vi "recordset get field names.vi"(8 "error in (no error)":errorcluster, 11 "recordset in":refnum<k7>) -> (0 "error out":errorcluster, 2 "field names":string[](array[string]), 3 "recordset out":refnum<k7>)   [LabVIEW 2020, in "ADODB.lvlib"]
uses:
  ADODB.lvlib
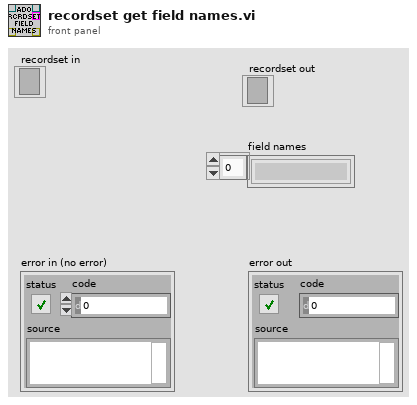
[diagram p1: front panel]
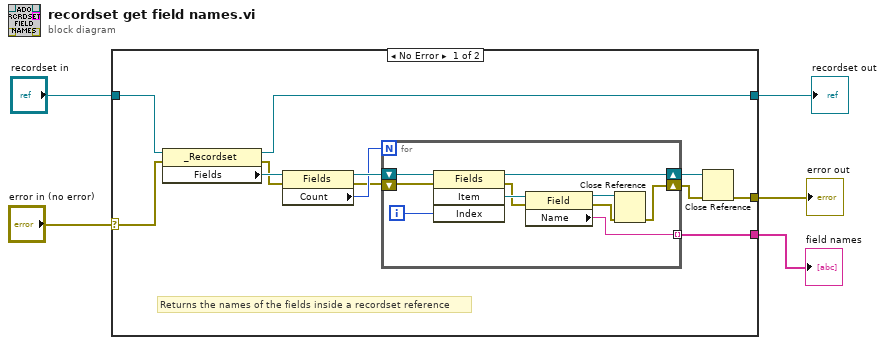
[diagram p0: block diagram]
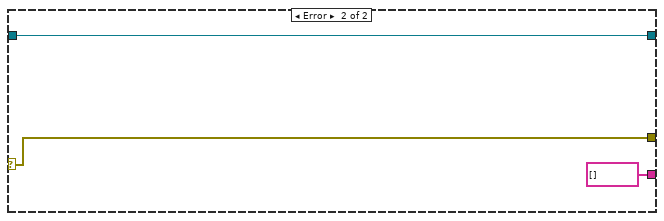
[diagram p2: hidden frame]
diagram:
  n1 = case shown="No Error" "error in (no error)" {
    selector: "error in (no error)" -> [w7 w30]
    tunnel: "recordset in" -> [w17 w28]
    tunnel: [w12 w28] -> w4
    tunnel: [w8 w30] -> w3
    tunnel: [w6 string[] []] -> w1
    frame No Error {
      # "Returns the names of the fields inside a recordset reference"
      n2 = property class="_Recordset"(reference=w17, error in=w7) -> (reference out=w12:refnum<k7>, error out=w11:errorcluster, "Fields"=w16:refnum<k7>)
      n3 = property class="Fields"(reference=w16, error in=w11) -> (reference out=w15:refnum<k7>, error out=w10:errorcluster, "Count"=w14:i32)
      n4 = for {
        N: w14 -> [_]
        tunnel: [w24] -> w6 mode=indexing
        shift-right: [w22] -> w13
        shift-left: w15 -> [w27]
        shift-right: [w18] -> w9
        shift-left: w10 -> [w21]
        i -> [w26]
        n5 = invoke class="Fields" method="Item"(reference=w27, error in=w21, "Index"=w26) -> (reference out=w22:refnum<k7>, error out=w20:errorcluster, "Item"=w25:refnum<k7>)  [unwired: 1 in, 1 out]
        n6 = property class="Field"(reference=w25, error in=w20) -> (reference out=w23:refnum<k7>, error out=w19:errorcluster, "Name"=w24:string)
        n7 = Close Reference(reference=w23, error in (no error)=w19) -> (error out=w18:errorcluster)
      }
      n8 = Close Reference(reference=w13, error in (no error)=w9) -> (error out=w8:errorcluster)
    }
    frame Error {
    }
  }
  "recordset out" <- w4
  "error out" <- w3
  "field names" <- w1
